vi "ETH_3 Main.vi"(8 "error in":errorcluster, 10 "data in":string, 11 "ETH3-Q":refnum<queue>) -> (0 "error out":errorcluster)   [LabVIEW 2022 SP3]
uses:
  6D_Global.vi
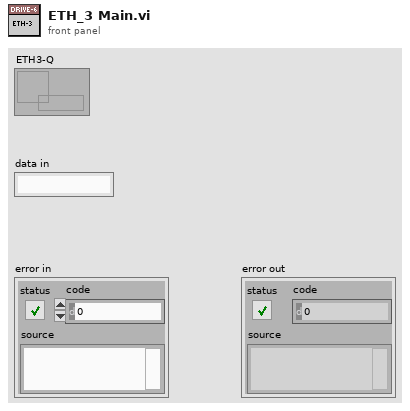
[diagram p1: front panel]
types:
  T1 = cluster{"Run ACK":dbl, "RDR":dbl, "Sector":dbl, "Halls Speed":dbl, "Mode":dbl, "Voltage Speed":dbl, "Direction":dbl, "IDC":dbl, "Movable average":dbl, "VDC":dbl}
  T2 = cluster{"Run ACK":bool, "RDR":dbl, "Sector":dbl, "Halls Speed":dbl, "Mode":bool, "Voltage Speed":dbl, "Direction":string, "IDC":dbl, "Movable average":dbl, "VDC":dbl}
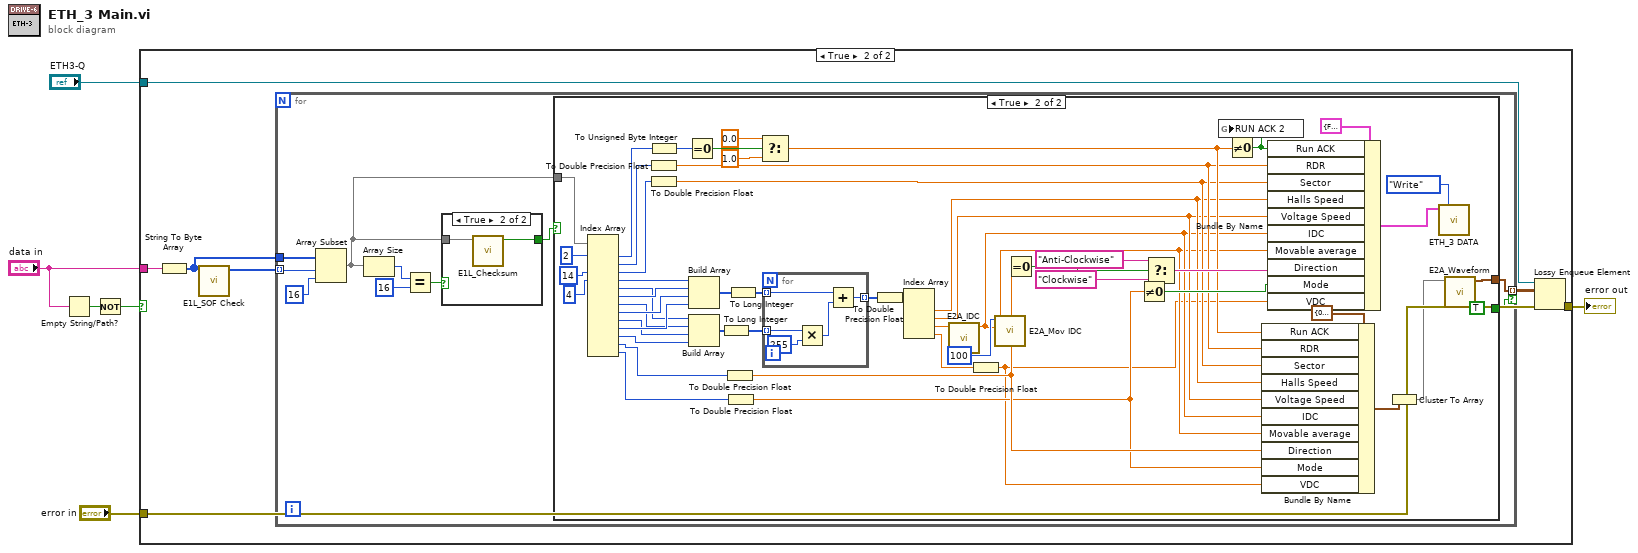
[diagram p0: block diagram]
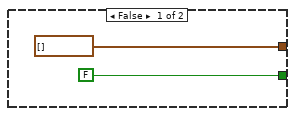
[diagram p3: hidden frame]
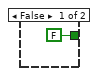
[diagram p4: hidden frame]
diagram:
  n1 = Empty String/Path?(string/path="data in") -> (empty?=w6:bool)
  n2 = Not(x=w6) -> (.not. x?=w5:bool)
  n3 = case shown="True" w5 {
    tunnel: "data in" -> [_ w14]
    tunnel: "ETH3-Q" -> [_ w10]
    tunnel: "error in" -> [w7 w9]
    tunnel: [w7 w8] -> w1
    frame False {
    }
    frame True {
      n4 = String To Byte Array(string=w14) -> (unsigned byte array=w12:u8[])
      n5 = call "E1L_SOF Check.vi"("Bytes data in"=w12) -> ("index of passed smpl"=w13:i32[])  [unwired: 8 in, 2 out]
      n6 = for {
        tunnel: w13 -> [w21] mode=indexing
        tunnel: w12 -> [w20]
        tunnel: [w17] -> w11 mode=indexing if=w15
        n7 = Array Subset(array=w20, index=w21, length=16) -> (w18:u8[])
        n8 = Array Size(array=w18) -> (size(s)=w23:i32)
        n9 = Equal?(x=w23, y=16) -> (x = y?=w19:bool)
        n10 = case shown="True" w19 {
          tunnel: w18 -> [_ w88]
          tunnel: [FALSE ("Checksum") w87] -> w16
          frame False {
          }
          frame True {
            n11 = call "E1L_Checksum.vi"("Data"=w88) -> ("Checksum"=w87:bool)  [unwired: 10 in]
          }
        }
        n12 = case shown="True" w16 {
          tunnel: w18 -> [_ w73]
          tunnel: [waveform(dbl)[] [] ("WF out") w70] -> w17
          tunnel: [FALSE TRUE] -> w15
          frame False {
          }
          frame True {
            n13 = Index Array(array=w73, index #1=2 ("index"), index #3=14 ("index"), index #4=4 ("index")) -> (element #1=w78:u8, element #2=w66:u8, element #3=w63:u8, element #4=w62:u8, element #5=w58:u8, element #6=w61:u8, element #7=w57:u8, element #8=w60:u8, element #9=w56:u8, element #10=w59:u8, element #11=w55:u8, element #12=w28:u8, element #13=w27:u8)  [unwired: 10 in]
            n14 = To Unsigned Byte Integer(number=w78) -> (unsigned 8bit integer=w79:u8)
            n15 = To Double Precision Float(number=w66) -> (double precision float=w40:dbl)
            n16 = To Double Precision Float(number=w63) -> (double precision float=w39:dbl)
            n17 = Equal To 0?(x=w79) -> (x = 0?=w80:bool)
            n18 = Build Array(w62, w61, w60, w59) -> (w54:u8[])
            n19 = Build Array(w58, w57, w56, w55) -> (w53:u8[])
            n20 = To Long Integer(number=w53) -> (32bit integer=w51:i32[])
            n21 = To Double Precision Float(number=w28) -> (double precision float=w34:dbl)
            n22 = To Double Precision Float(number=w27) -> (double precision float=w33:dbl)
            n23 = To Long Integer(number=w54) -> (32bit integer=w52:i32[])
            n24 = Select(t=0.0, s=w80, f=1.0) -> (s? t:f=w41:dbl)
            n25 = for {
              tunnel: [w84] -> w77 mode=indexing
              tunnel: w52 -> [w82] mode=indexing
              tunnel: w51 -> [w81] mode=indexing
              n26 = Multiply(x=w81, y=255) -> (x*y=w85:i32)
              n27 = Add(x=w82, y=w85) -> (x+y=w84:i32)
            }
            n28 = To Double Precision Float(number=w77) -> (double precision float=w76:dbl[])
            n29 = Index Array(array=w76) -> (element #1=w38:dbl, element #2=w37:dbl, element #3=w50:dbl, element #4=w29:dbl)  [unwired: 4 in]
            n30 = call "E2A_IDC.vi"("IDC in"=w50) -> ("IDC out"=w36:dbl)  [unwired: 10 in]
            n31 = To Double Precision Float(number=w29) -> (double precision float=w30:dbl)
            n32 = call "E2A_Mov IDC.vi"("Idc"=w36, "SampleSize"=100) -> ("Mean"=w35:dbl)  [unwired: 9 in]
            n33 = Equal To 0?(x=w34) -> (x = 0?=w49:bool)
            n34 = Not Equal To 0?(x=w33) -> (x != 0?=w45:bool)
            n35 = Select(t="Anti-Clockwise" ("Direction"), s=w49, f="Clockwise" ("Direction")) -> (s? t:f=w48:string)
            n36 = Not Equal To 0?(x=w41) -> (x != 0?=w67:bool)
            n37 = global write "6D_Global.vi" "RUN ACK 2"(w67) -> ()
            n38 = Bundle By Name(cluster=T1 {"Run ACK"=0.0, "RDR"=0.0, "Sector"=0.0, "Halls Speed"=0.0, "Mode"=0.0, "Voltage Speed"=0.0, "Direction"=0.0, "IDC"=0.0, "Movable average"=0.0, "VDC"=0.0} ("output cluster"), "Run ACK"=w41, "RDR"=w40, "Sector"=w39, "Halls Speed"=w38, "Voltage Speed"=w37, "IDC"=w36, "Movable average"=w35, "Direction"=w34, "Mode"=w33, "VDC"=w30) -> (w43:T1)
            n39 = Bundle By Name(cluster=T2 {"Run ACK"=FALSE, "RDR"=0.0, "Sector"=0.0, "Halls Speed"=0.0, "Mode"=TRUE, "Voltage Speed"=0.0, "Direction"="", "IDC"=0.0, "Movable average"=0.0, "VDC"=0.0} ("Motor Feedback"), "Run ACK"=w67, "RDR"=w40, "Sector"=w39, "Halls Speed"=w38, "Voltage Speed"=w37, "IDC"=w36, "Movable average"=w35, "Direction"=w48, "Mode"=w45, "VDC"=w30) -> (w32:T2)
            n40 = Cluster To Array(cluster=w43) -> (array=w42:dbl[])
            n41 = call "ETH_3 DATA.vi"("Enum"=enum16{"Read", "Write"}."Write", "ETH 3"=w32) -> ()  [unwired: 8 in, 2 out]
            n42 = call "E2A_Waveform.vi"("Data in"=w42) -> ("WF out"=w70:waveform(dbl)[])  [unwired: 10 in]
          }
        }
      }
      n43 = Lossy Enqueue Element(queue=w10, element=w11, error in (no error)=w9) -> (error out=w8:errorcluster)  [unwired: 3 out]
    }
  }
  "error out" <- w1
